vi "ProgressBar setCaption.vi"(8 "error in (no error)":errorcluster, 10 "newCaption":string, 11 "ProgressBar in":refnum<class "ProgressBar.lvclass">) -> (0 "error out":errorcluster, 3 "ProgressBar out":refnum<class "ProgressBar.lvclass">)   [LabVIEW 2018, in "ProgressBar.lvclass"]
uses:
  ProgressBar.lvclass
  ProgressBar.lvclass/ProgressBar.ctl
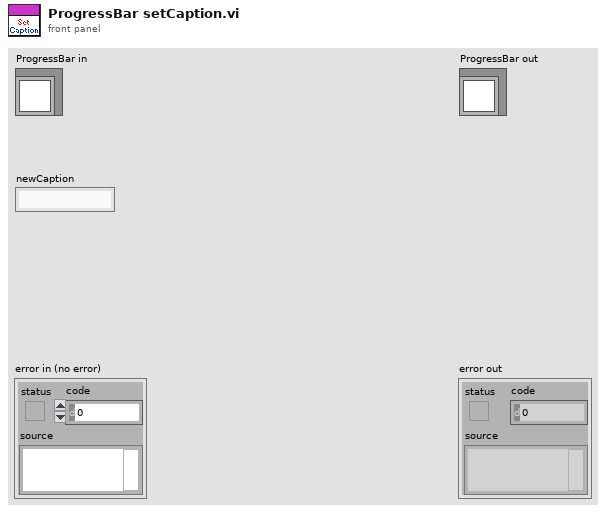
[diagram p1: front panel]
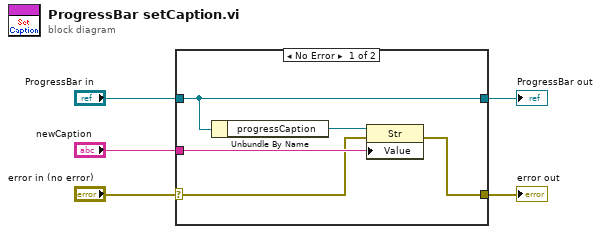
[diagram p0: block diagram]
diagram:
  n1 = case shown="No Error" "error in (no error)" {
    selector: "error in (no error)" -> [w7 w12]
    tunnel: [w6 w12] -> w4
    tunnel: [w10 w11] -> w2
    tunnel: "ProgressBar in" -> [w10 w11]
    tunnel: "newCaption" -> [w8 _]
    frame No Error {
      n2 = Unbundle By Name(w10) -> ("progressCaption"=w9:refnum<vi>)
      n3 = property class="Str"(reference=w9, error in=w7, "Value"=w8) -> (error out=w6:errorcluster)  [unwired: 1 out]
    }
    frame Error {
    }
  }
  "error out" <- w4
  "ProgressBar out" <- w2
